vi "least square linear interpolation.vi"(10 "X":dbl[](array[numeric])=[1.0, 2.0, 3.0], 11 "Y":dbl[](array[numeric])=[-1.0, -2.0, -3.0]) -> (0 "mean Y":dbl, 1 "intercept":dbl=-0.0, 2 "slope":dbl=-1.0, 3 "mean X":dbl)   [LabVIEW 2021]
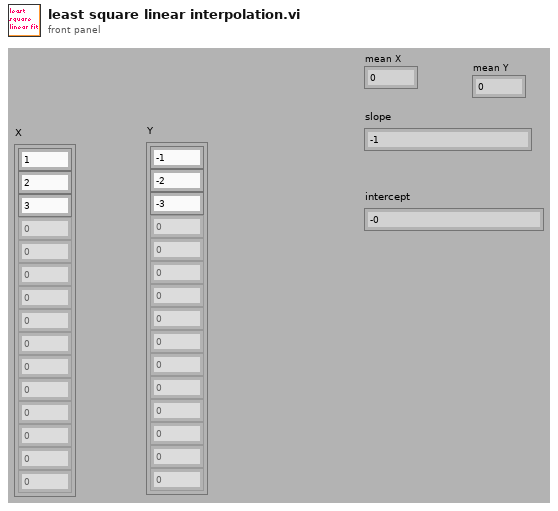
[diagram p1: front panel]
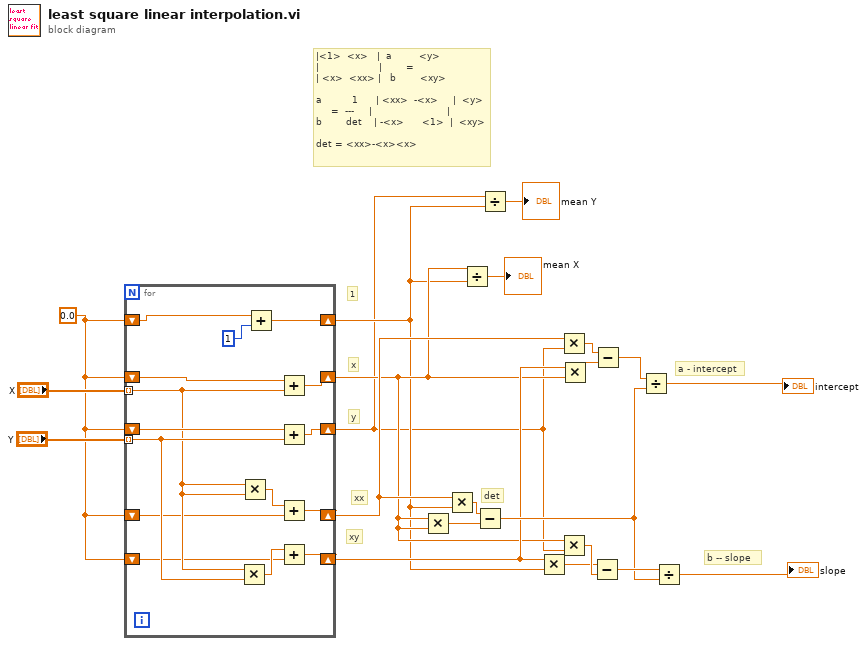
[diagram p0: block diagram]
diagram:
  w19 = 0.0
  # "b -- slope"
  # "a - intercept"
  # "|<1>  <x>   |  a         <y>\n|                    |        =   \n| <x>  <xx> |   b        <xy> \n\na          1      | <xx>  -<x>     |  <y>\n     =  ---     |                         |\nb        det    | -<x>      <1>  |  <xy>\n\ndet = <xx>-<x><x>"
  # "det"
  # "xy"
  # "xx"
  # "y"
  # "x"
  # "1"
  n1 = for {
    shift-right: [w36] -> w2
    shift-left: w19 -> [w35]
    shift-right: [w32] -> w5
    shift-left: w19 -> [w33]
    tunnel: "X" -> [w28] mode=indexing
    tunnel: "Y" -> [w29] mode=indexing
    shift-right: [w30] -> w1
    shift-left: w19 -> [w31]
    shift-right: [w24] -> w9
    shift-left: w19 -> [w25]
    shift-right: [w22] -> w7
    shift-left: w19 -> [w23]
    n2 = Multiply(x=w28, y=w29) -> (x*y=w26:dbl)
    n3 = Multiply(x=w28, y=w28) -> (x*y=w27:dbl)
    n4 = Add(x=w35, y=1) -> (x+y=w36:dbl)
    n5 = Add(x=w33, y=w28) -> (x+y=w32:dbl)
    n6 = Add(x=w31, y=w29) -> (x+y=w30:dbl)
    n7 = Add(x=w27, y=w25) -> (x+y=w24:dbl)
    n8 = Add(x=w26, y=w23) -> (x+y=w22:dbl)
  }
  n9 = Multiply(x=w5, y=w5) -> (x*y=w18:dbl)
  n10 = Multiply(x=w9, y=w2) -> (x*y=w8:dbl)
  n11 = Divide(x=w5, y=w2) -> (x/y=→"mean X":dbl)
  n12 = Subtract(x=w8, y=w18) -> (x-y=w12:dbl)
  n13 = Divide(x=w1, y=w2) -> (x/y=→"mean Y":dbl)
  n14 = Multiply(x=w7, y=w2) -> (x*y=w6:dbl)
  n15 = Multiply(x=w9, y=w1) -> (x*y=w17:dbl)
  n16 = Multiply(x=w5, y=w1) -> (x*y=w14:dbl)
  n17 = Multiply(x=w7, y=w5) -> (x*y=w16:dbl)
  n18 = Subtract(x=w6, y=w14) -> (x-y=w13:dbl)
  n19 = Subtract(x=w17, y=w16) -> (x-y=w15:dbl)
  n20 = Divide(x=w15, y=w12) -> (x/y=→"intercept":dbl)
  n21 = Divide(x=w13, y=w12) -> (x/y=→"slope":dbl)
